vi "Set Stop Time.vi"(6 "New Stop Time":timestamp format="%<%x %.3X>T", 8 "error in (no error)":errorcluster, 10 "Use Current Time? (T)":bool=TRUE, 11 "Time Entries in":refnum<class "Time Entries.lvclass">) -> (0 "error out":errorcluster, 2 "Display":string[](array[string]) caption="Initial Display", 3 "Time Entries out":refnum<class "Time Entries.lvclass">)   [LabVIEW 2020, in "Time Entries.lvclass"]
doc: "Adds either the Current Time (Default) or the time specified in the New Stop Time as the stop time for the time entry.\n\n04/2025 Erich Schlieper"
uses:
  Time Entries.lvclass
  Time Entries.lvclass/Time Entries.ctl
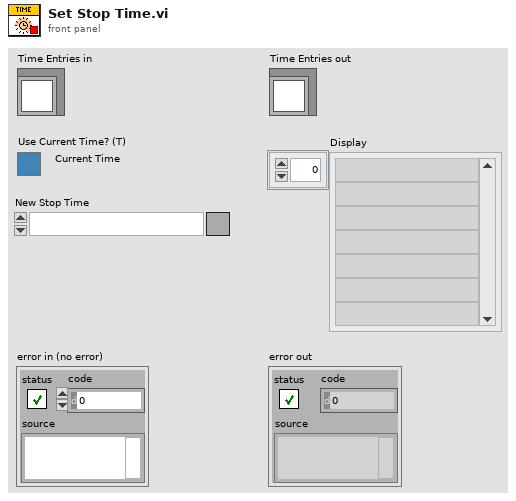
[diagram p1: front panel]
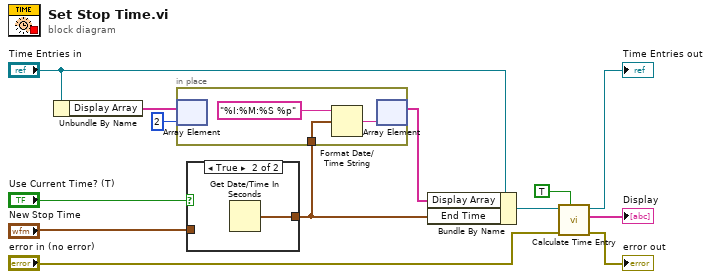
[diagram p0: block diagram]
diagram:
  n1 = Unbundle By Name("Time Entries in") -> ("Display Array"=w4:string[])
  n2 = case shown="True" "Use Current Time? (T)" {
    tunnel: [w14 w15] -> w2
    tunnel: "New Stop Time" -> [w14 _]
    frame False {
    }
    frame True {
      n3 = Get Date/Time In Seconds() -> (seconds since 1Jan1904=w15:timestamp)
    }
  }
  n4 = in-place {
    in-place-border: w2 -> [w17]
    n5 = in-place-array #1(w4, 2) -> ()  [unwired: 1 out]
    n6 = Format Date/Time String(time format string (%c)="%I:%M:%S %p", seconds (now)=w17) -> (date/time string=w16:string)  [unwired: 1 in]
    n7 = in-place-array #1(w16) -> (w1:string[])  [unwired: 1 out]
  }
  n8 = Bundle By Name(cluster="Time Entries in", "Display Array"=w1, "End Time"=w2) -> (w6:refnum<class "Time Entries.lvclass">)
  n9 = call-dynamic "Calculate Time Entry.vi"("Recalculate Override (F)"=TRUE, "error in (no error)"="error in (no error)", "Time Entries in"=w6) -> ("error out"=→"error out":errorcluster, "Display"=→"Display":string[], "Time Entries out"=→"Time Entries out":refnum<class "Time Entries.lvclass">)  [unwired: 6 in]
